vi "Create Data Entry for Log.vi"(6 "Units":string, 8 "error in (no error)":errorcluster, 9 "Sensor Name":string, 10 "Data In":dbl, 11 "MWWL Verification in":refnum<class "MWWL Verification.lvclass">) -> (0 "error out":errorcluster, 3 "MWWL Verification out":refnum<class "MWWL Verification.lvclass">)   [LabVIEW 2018, in "MWWL Verification.lvlib" / "MWWL Verification.lvclass"]
uses:
  MWWL Verification.lvclass
  C:/Program Files (x86)/National Instruments/LabVIEW 2018/vi.lib/ActorFramework/Actor/Actor.lvclass
  Type Defs/Data Record Control.ctl
  <vilib>/ActorFramework/Actor/Actor.lvclass/Actor.ctl
  <vilib>/ActorFramework/Message Enqueuer/Message Enqueuer.lvclass/Message Enqueuer.ctl
  MWWL Verification Messages/Send Value to Datalogger Msg/Send Value to Datalogger Msg.lvclass/Send Value to Datalogger Msg.ctl
  <vilib>/ActorFramework/Message Enqueuer/Init from Existing Queue.vi
  <vilib>/ActorFramework/Message Enqueuer/Enqueue.vi
  MWWL Verification Messages/Send Value to Datalogger Msg/Send Value to Datalogger Msg.lvclass
  C:/Program Files (x86)/National Instruments/LabVIEW 2018/vi.lib/ActorFramework/Message/Message.lvclass
  <vilib>/ActorFramework/Message Priority Queue/Priority Enqueue.vi
  <vilib>/ActorFramework/Message Enqueuer/Message Enqueuer.lvclass
  <vilib>/ActorFramework/Actor/Actor.lvclass
  MWWL Verification.lvlib
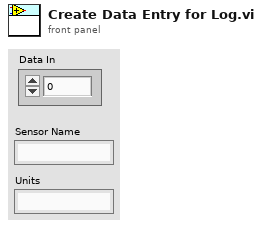
[diagram p1: front panel]
types:
  T1 = typedef "MWWL Verification.lvlib/Data Record Control.ctl" = cluster{"Timestamp":string, "Sensor Name":string, "Data (string)":string, "Units":string}
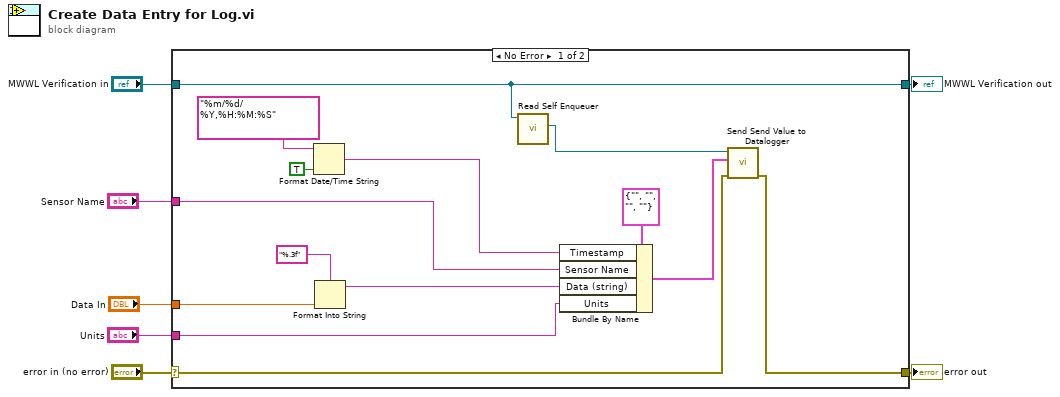
[diagram p0: block diagram]
diagram:
  n1 = case shown="No Error" "error in (no error)" {
    selector: "error in (no error)" -> [w9 w23]
    tunnel: [w8 w23] -> w6
    tunnel: [w17 w22] -> w4
    tunnel: "MWWL Verification in" -> [w17 w22]
    tunnel: "Data In" -> [w21 _]
    tunnel: "Sensor Name" -> [w12 _]
    tunnel: "Units" -> [w10 _]
    frame No Error {
      n2 = Format Date/Time String(time format string (%c)="%m/%d/%Y,%H:%M:%S", UTC format=TRUE) -> (date/time string=w13:string)  [unwired: 1 in]
      n3 = Format Into String(format string="%.3f", w21) -> (resulting string=w11:string)  [unwired: 2 in, 1 out]
      n4 = call <vilib>:"Read Self Enqueuer.vi"("Actor"=w17) -> ("Self Enqueuer"=w16:refnum<class "Message Enqueuer.lvclass">)  [unwired: 10 in]
      n5 = Bundle By Name(cluster=T1 {"Timestamp"="", "Sensor Name"="", "Data (string)"="", "Units"=""} ("Data Record"), "Timestamp"=w13, "Sensor Name"=w12, "Data (string)"=w11, "Units"=w10) -> (w14:T1)
      n6 = call "Send Send Value to Datalogger.vi"("error in (no error)"=w9, "Data Record"=w14, "Message Enqueuer in"=w16) -> ("error out"=w8:errorcluster)  [unwired: 7 in, 1 out]
    }
    frame Error {
    }
  }
  "error out" <- w6
  "MWWL Verification out" <- w4
